vi "replace_ego_pose.vi"(4 "error in":errorcluster, 5 "Ego pose":T2={"angular velocity"=[0.0, 0.0, 0.0], "velocity"=[0.0, 0.0, 0.0], "steering_direction"=0.0, "position"=[0.0, 0.0, 0.0], "orientation YPR"={"yaw"=0.001, "pitch"=0.0, "roll"=0.0}} {"orientation YPR"."yaw" min=0.0 step=0.1 format="%#_5f"; "steering_direction" format="%#_13g"}, 6 "Frames":T1(array[cluster]), 7 "Frame number":i32) -> (0 "error out":errorcluster, 3 "Frame":string)   [LabVIEW 2019]
doc: "Replace the pose for the ego vehicle on a specific frame and outputs the JSON corresponding to the frame with the new settings."
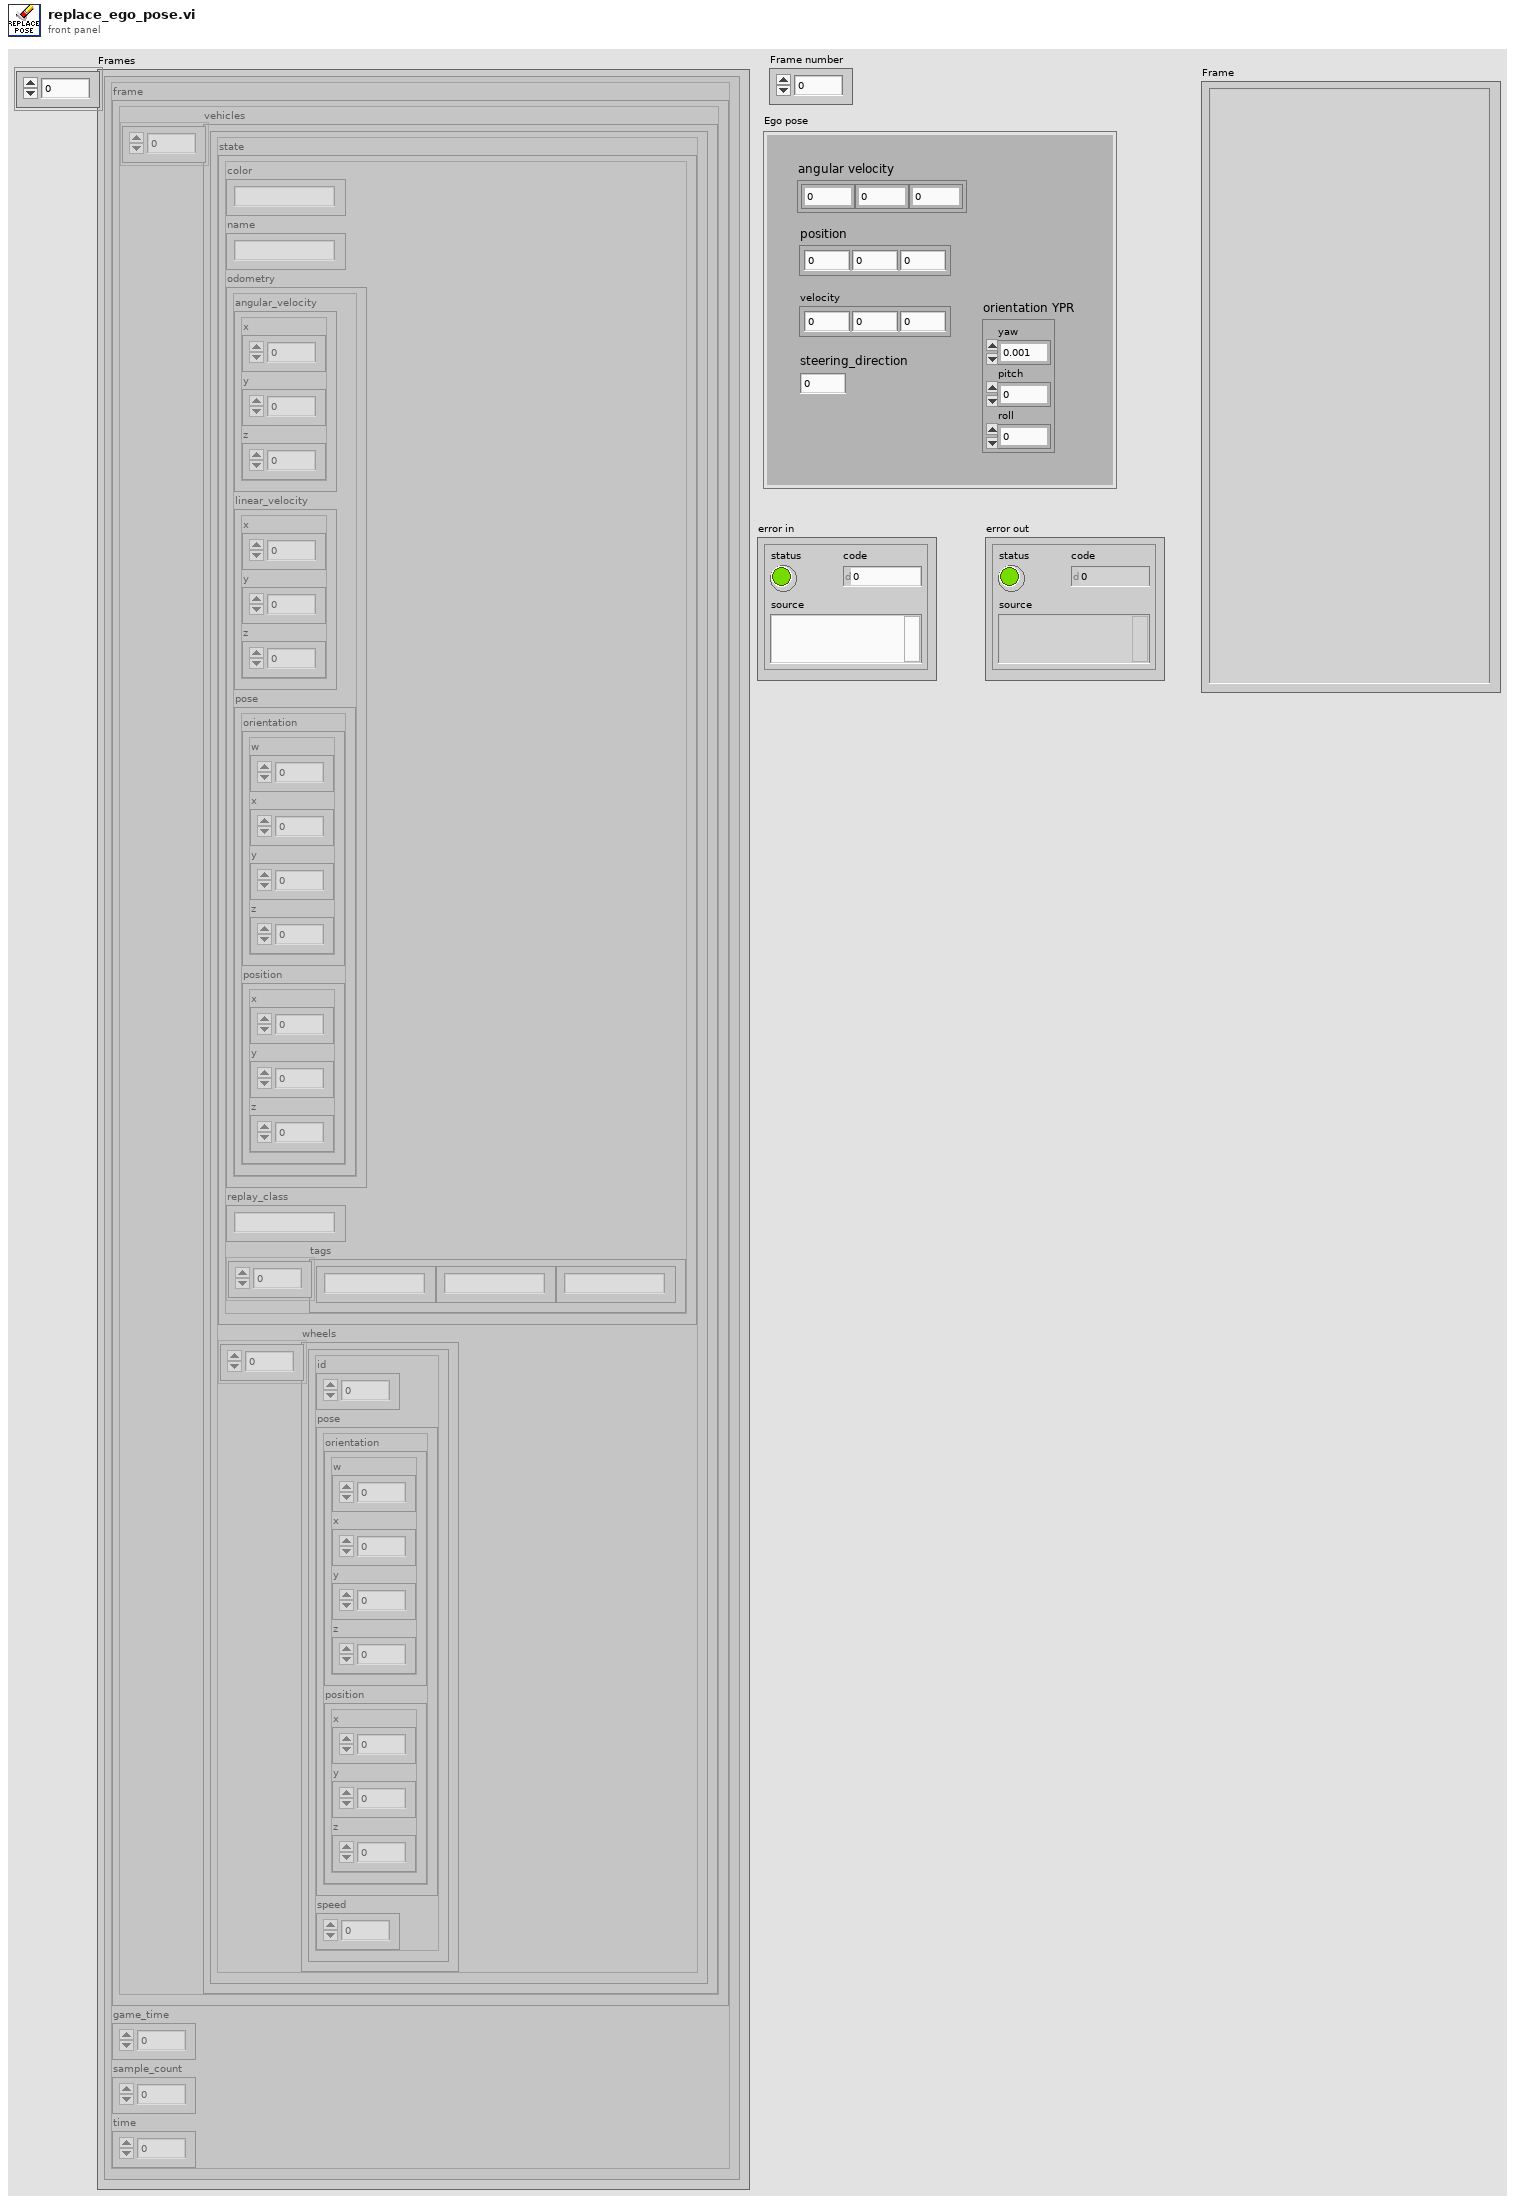
[diagram p1: front panel]
types:
  T1 = cluster{"frame":cluster{"vehicles":cluster{"state":cluster{"color":string, "name":string, "odometry":cluster{"angular_velocity":cluster{"x":dbl, "y":dbl, "z":dbl}, "linear_velocity":cluster{"x":dbl, "y":dbl, "z":dbl}, "pose":cluster{"orientation":cluster{"w":dbl, "x":dbl, "y":dbl, "z":dbl}, "position":cluster{"x":dbl, "y":dbl, "z":dbl}}}, "replay_class":string, "tags":string[]}, "wheels":cluster{"id":i32, "pose":cluster{"orientation":cluster{"w":dbl, "x":dbl, "y":dbl, "z":dbl}, "position":cluster{"x":dbl, "y":dbl, "z":dbl}}, "speed":dbl}[]}[]}, "game_time":dbl, "sample_count":dbl, "time":dbl}[]
  T2 = cluster{"angular velocity":dbl[], "velocity":dbl[], "steering_direction":dbl, "position":dbl[], "orientation YPR":cluster{"yaw":dbl, "pitch":dbl, "roll":dbl}}
  T3 = cluster{"frame":cluster{"vehicles":cluster{"state":cluster{"color":string, "name":string, "odometry":cluster{"angular_velocity":cluster{"x":dbl, "y":dbl, "z":dbl}, "linear_velocity":cluster{"x":dbl, "y":dbl, "z":dbl}, "pose":cluster{"orientation":cluster{"w":dbl, "x":dbl, "y":dbl, "z":dbl}, "position":cluster{"x":dbl, "y":dbl, "z":dbl}}}, "replay_class":string, "tags":string[]}, "wheels":cluster{"id":i32, "pose":cluster{"orientation":cluster{"w":dbl, "x":dbl, "y":dbl, "z":dbl}, "position":cluster{"x":dbl, "y":dbl, "z":dbl}}, "speed":dbl}[]}[]}, "game_time":dbl, "sample_count":dbl, "time":dbl}
  T4 = cluster{"state":cluster{"color":string, "name":string, "odometry":cluster{"angular_velocity":cluster{"x":dbl, "y":dbl, "z":dbl}, "linear_velocity":cluster{"x":dbl, "y":dbl, "z":dbl}, "pose":cluster{"orientation":cluster{"w":dbl, "x":dbl, "y":dbl, "z":dbl}, "position":cluster{"x":dbl, "y":dbl, "z":dbl}}}, "replay_class":string, "tags":string[]}, "wheels":cluster{"id":i32, "pose":cluster{"orientation":cluster{"w":dbl, "x":dbl, "y":dbl, "z":dbl}, "position":cluster{"x":dbl, "y":dbl, "z":dbl}}, "speed":dbl}[]}[]
  T5 = cluster{"id":i32, "pose":cluster{"orientation":cluster{"w":dbl, "x":dbl, "y":dbl, "z":dbl}, "position":cluster{"x":dbl, "y":dbl, "z":dbl}}, "speed":dbl}[]
  T6 = cluster{"angular_velocity 2":dbl, "angular_velocity 2":dbl, "angular_velocity 2":dbl}
  T7 = cluster{"state":cluster{"color":string, "name":string, "odometry":cluster{"angular_velocity":cluster{"x":dbl, "y":dbl, "z":dbl}, "linear_velocity":cluster{"x":dbl, "y":dbl, "z":dbl}, "pose":cluster{"orientation":cluster{"w":dbl, "x":dbl, "y":dbl, "z":dbl}, "position":cluster{"x":dbl, "y":dbl, "z":dbl}}}, "replay_class":string, "tags":string[]}, "wheels":cluster{"id":i32, "pose":cluster{"orientation":cluster{"w":dbl, "x":dbl, "y":dbl, "z":dbl}, "position":cluster{"x":dbl, "y":dbl, "z":dbl}}, "speed":dbl}[]}
  T8 = cluster{cluster{"state":cluster{"color":string, "name":string, "odometry":cluster{"angular_velocity":cluster{"x":dbl, "y":dbl, "z":dbl}, "linear_velocity":cluster{"x":dbl, "y":dbl, "z":dbl}, "pose":cluster{"orientation":cluster{"w":dbl, "x":dbl, "y":dbl, "z":dbl}, "position":cluster{"x":dbl, "y":dbl, "z":dbl}}}, "replay_class":string, "tags":string[]}, "wheels":cluster{"id":i32, "pose":cluster{"orientation":cluster{"w":dbl, "x":dbl, "y":dbl, "z":dbl}, "position":cluster{"x":dbl, "y":dbl, "z":dbl}}, "speed":dbl}[]}[]}
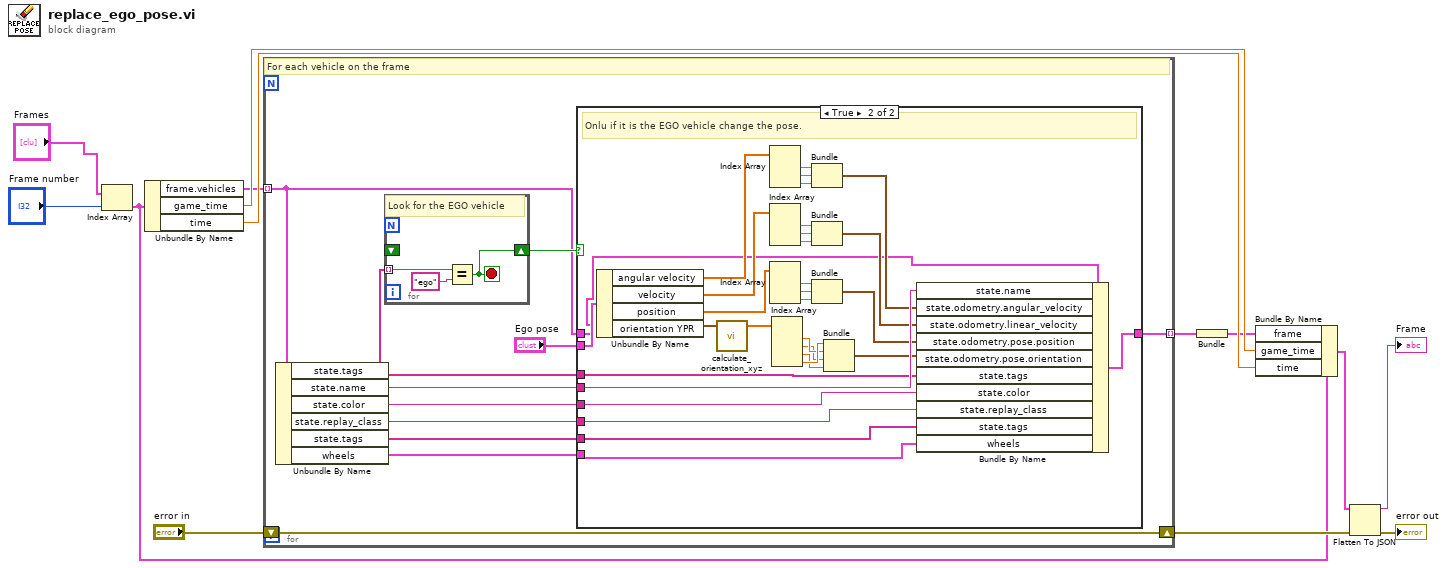
[diagram p0: block diagram]
diagram:
  n1 = Index Array(array="Frames", index="Frame number") -> (element=w4:T3)
  n2 = Unbundle By Name(w4) -> ("frame.vehicles"=w8:T4, "game_time"=w9:dbl, "time"=w10:dbl)
  n3 = for {
    tunnel: w8 -> [w22] mode=indexing
    shift-right: [w21] -> w13
    shift-left: "error in" -> [w21]
    tunnel: [w19] -> w3 mode=indexing
    # "For each vehicle on the frame"
    n4 = Unbundle By Name(w22) -> ("state.tags"=w24:string[], "state.name"=w18:string, "state.color"=w17:string, "state.replay_class"=w16:string, "state.tags"=w15:string[], "wheels"=w14:T5)
    n5 = for {
      tunnel: w24 -> [w59] mode=indexing
      shift-right: [w57] -> w23
      shift-left: _ -> [_]
      stop <- w57 stop-if-true
      # "Look for the EGO vehicle"
      n6 = Equal?(x=w59, y="ego") -> (x = y?=w57:bool)
    }
    n7 = case shown="True" w23 {
      tunnel: w24 -> [_ w37]
      tunnel: w18 -> [_ w55]
      tunnel: w22 -> [w25 w30]
      tunnel: [w25 w36] -> w19
      tunnel: "Ego pose" -> [_ w56]
      tunnel: w17 -> [_ w29]
      tunnel: w16 -> [_ w28]
      tunnel: w15 -> [_ w27]
      tunnel: w14 -> [_ w26]
      frame False {
        # "Send the values without change for other vehicles"
      }
      frame True {
        # "Onlu if it is the EGO vehicle change the pose."
        n8 = Unbundle By Name(w56) -> ("angular velocity"=w53:dbl[], "velocity"=w45:dbl[], "position"=w42:dbl[], "orientation YPR"=w54:cluster{"yaw":dbl, "pitch":dbl, "roll":dbl})
        n9 = call "calculate_orientation_xyz.vi"("orientation YPR"=w54) -> ("pose"=w43:dbl[])  [unwired: 4 in]
        n10 = Index Array(array=w53) -> (element #1=w52:dbl, element #2=w51:dbl, element #3=w50:dbl)  [unwired: 3 in]
        n11 = Index Array(array=w45) -> (element #1=w46:dbl, element #2=w47:dbl, element #3=w48:dbl)  [unwired: 3 in]
        n12 = Index Array(array=w42) -> (element #1=w41:dbl, element #2=w40:dbl, element #3=w39:dbl)  [unwired: 3 in]
        n13 = Index Array(array=w43) -> (element #1=w33:dbl, element #2=w32:dbl, element #3=w31:dbl, element #4=w34:dbl)  [unwired: 4 in]
        n14 = Bundle("angular_velocity 2"=w52, "angular_velocity 2"=w51, "angular_velocity 2"=w50) -> (w49:T6)  [unwired: 1 in]
        n15 = Bundle("angular_velocity 2"=w46, "angular_velocity 2"=w47, "angular_velocity 2"=w48) -> (w44:T6)  [unwired: 1 in]
        n16 = Bundle("angular_velocity 2"=w41, "angular_velocity 2"=w40, "angular_velocity 2"=w39) -> (w38:T6)  [unwired: 1 in]
        n17 = Bundle(w34, w33, w32, w31) -> (w35:cluster{dbl, dbl, dbl, dbl})  [unwired: 1 in]
        n18 = Bundle By Name(cluster=w30, "state.name"=w55, "state.odometry.angular_velocity"=w49, "state.odometry.linear_velocity"=w44, "state.odometry.pose.position"=w38, "state.odometry.pose.orientation"=w35, "state.tags"=w37, "state.color"=w29, "state.replay_class"=w28, "state.tags"=w27, "wheels"=w26) -> (w36:T7)
      }
    }
  }
  n19 = Bundle(w3) -> (w2:T8)  [unwired: 1 in]
  n20 = Bundle By Name(cluster=w4, "frame"=w2, "game_time"=w9, "time"=w10) -> (w11:T3)
  n21 = Flatten To JSON(anything=w11, error in (no error)=w13) -> (JSON string=→"Frame":string, 11:→"error out":errorcluster)  [unwired: 1 in]
